vi "Apply Channel Range.vi"(8 "error in":errorcluster, 11 "4300 in":refnum<class "4300.lvclass">) -> (0 "error out":errorcluster, 3 "4300 out":refnum<class "4300.lvclass">)   [LabVIEW 2019, in "4300.lvlib" / "4300.lvclass"]
uses:
  Library/4300.lvclass
  C:/Users/Public/Documents/Development/builds/Instruments/AnalogInput.lvlibp/Library/AnalogInput.lvclass
  Library/4300.lvclass/4300.ctl
  builds/Instruments/AnalogInput.lvlibp/Accessors/GUI/Read Channel Names.vi
  builds/Instruments/AnalogInput.lvlibp/Accessors/Read Range.vi
  <vilib>/DAQmx/create/channels.llb/DAQmx Create Channel (AI-Voltage-Basic).vi
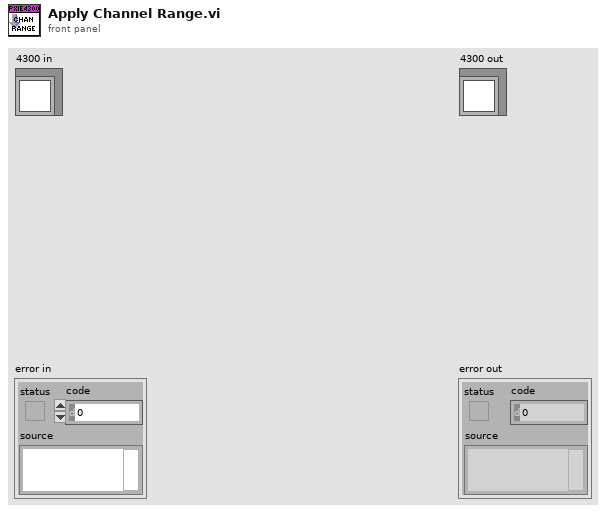
[diagram p1: front panel]
types:
  T1 = typedef "AnalogInput.lvlibp/AnalogInput.lvclass/Range.ctl" = cluster{"Max Value":dbl, "Min Value":dbl}
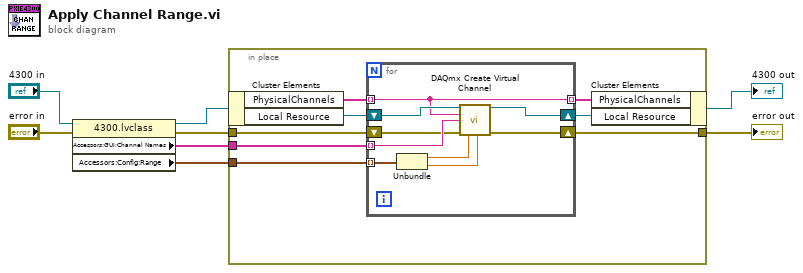
[diagram p0: block diagram]
diagram:
  n1 = property class="4300.lvclass"(reference="4300 in", error in="error in") -> (reference out=w6:refnum<class "4300.lvclass">, error out=w4:errorcluster, "Accessors:GUI:Channel Names"=w3:string[], "Accessors:Config:Range"=w2:T1[])
  n2 = in-place {
    in-place-border: w4 -> [w10]
    in-place-border: w3 -> [w12]
    in-place-border: w2 -> [w11]
    in-place-border: [w9] -> w1
    n3 = in-place-cluster #1(w6) -> ("PhysicalChannels"=w16:tag[], "Local Resource"=w14:refnum<k21>)
    n4 = for {
      tunnel: w16 -> [w23] mode=indexing
      tunnel: [w23] -> w15 mode=indexing
      shift-right: [w24] -> w13
      shift-left: w14 -> [w25]
      tunnel: w12 -> [w22] mode=indexing
      tunnel: w11 -> [w21] mode=indexing
      shift-right: [w18] -> w9
      shift-left: w10 -> [w17]
      n5 = Unbundle(w21) -> ("Max Value"=w20:dbl, "Min Value"=w19:dbl)
      n6 = call-poly <vilib>:"DAQmx Create Virtual Channel.vi"("task in"=w25, "maximum value"=w20, "minimum value"=w19, "physical channels"=w23, "name to assign"=w22, "error in"=w17) -> ("task out"=w24:refnum<k21>, "error out"=w18:errorcluster)  [unwired: 8 in]
    }
    n7 = in-place-cluster #1("PhysicalChannels"=w15, "Local Resource"=w13) -> (→"4300 out":refnum<class "4300.lvclass">)
  }
  "error out" <- w1
